vi "8.7.vi"() -> ()   [LabVIEW 2017]
panel:
  in  "element":dbl
  in  "in":dbl[](array[numeric])
  out "uit":dbl[](array[numeric])
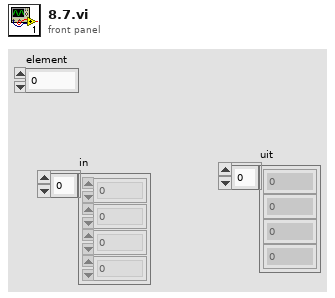
[diagram p1: front panel]
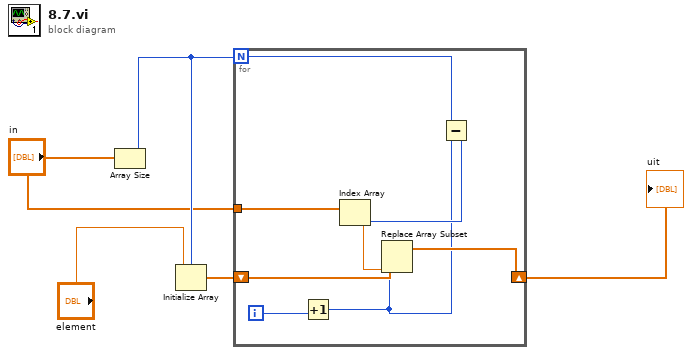
[diagram p0: block diagram]
diagram:
  n1 = Array Size(array="in") -> (size(s)=w4:i32)
  n2 = Initialize Array("element", w4) -> (w3:dbl[])
  n3 = for {
    N: w4 -> [w6]
    shift-right: [w12] -> w2
    shift-left: w3 -> [w13]
    tunnel: "in" -> [w11]
    i -> [w8]
    n4 = Increment(x=w8) -> (x+1=w7:i32)
    n5 = Subtract(x=w6, y=w7) -> (x-y=w10:i32)
    n6 = Index Array(array=w11, index=w10) -> (element=w9:dbl)
    n7 = Replace Array Subset(array=w13, new element=w9, index=w7) -> (w12:dbl[])
  }
  "uit" <- w2
